vi "Write Player Info.vi"(8 "error in (no error)":errorcluster, 10 "Player Info":T1={"Name"="", "Color Box"=0, "Gloat Phrase"="All your base are belong to us!!"}, 11 "Explorer in":refnum<class "Explorer.lvclass">) -> (0 "error out":errorcluster, 3 "Explorer out":refnum<class "Explorer.lvclass">)   [LabVIEW 2014, in "Explorer.lvclass"]
uses:
  Explorer.lvclass
  Player Info.ctl
  Runner.lvclass
  SquareBattle.lvclass
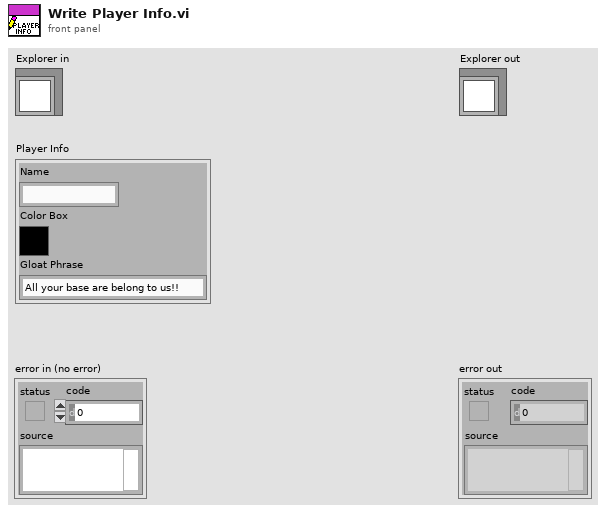
[diagram p1: front panel]
types:
  T1 = typedef "SquareBattle.lvclass/Player Info.ctl" = cluster{"Name":string, "Color Box":u32, "Gloat Phrase":string}
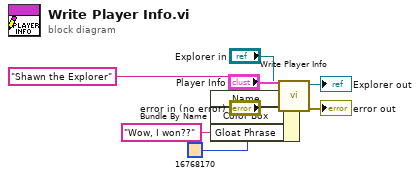
[diagram p0: block diagram]
diagram:
  n1 = Bundle By Name(cluster="Player Info", "Name"="Shawn the Explorer", "Color Box"=u32 16768170, "Gloat Phrase"="Wow, I won??") -> (w4:T1)
  n2 = call-parent "Write Player Info.vi"("error in (no error)"="error in (no error)", "Player Info"=w4, "Runner in"="Explorer in") -> ("error out"=→"error out":errorcluster, "Runner out"=→"Explorer out":refnum<class "Explorer.lvclass">)  [unwired: 7 in]
